vi "Untitled 1 (SubVI).vi"(7 "Comm":enum16{"Init", "Clear", "Update Data"}(ring), 8 "error in (no error)":errorcluster, 10 "Channels info":string[](array[string])=["燃烧室压力1\n[MPa]", "燃烧室压力1\n[MPa]"], 11 "ML Ref":refnum<vi>) -> (0 "error out":errorcluster)   [LabVIEW 2016]
uses:
  <vilib>/Utility/miscctls.llb/LVRowAndColumnTypeDef.ctl
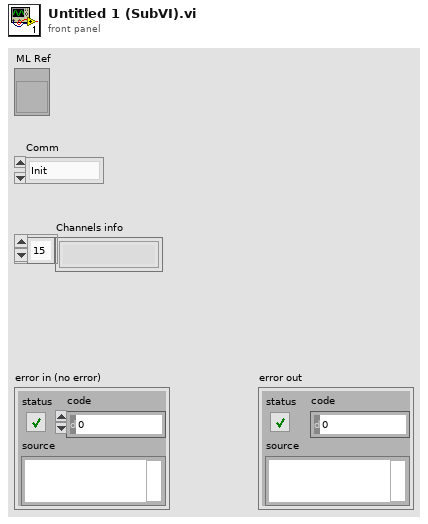
[diagram p1: front panel]
types:
  T1 = cluster{"Font Name":string, "Size":u16, "Bold":bool, "Italic":bool, "Underline":bool, "Strikeout":bool, u32}
  T2 = typedef "LVRowAndColumnTypeDef.ctl" = cluster{"Row":i32, "Column":i32}
  T3 = typedef "LVBoundsTypeDef.ctl" = cluster{"Width":u32, "Height":u32}
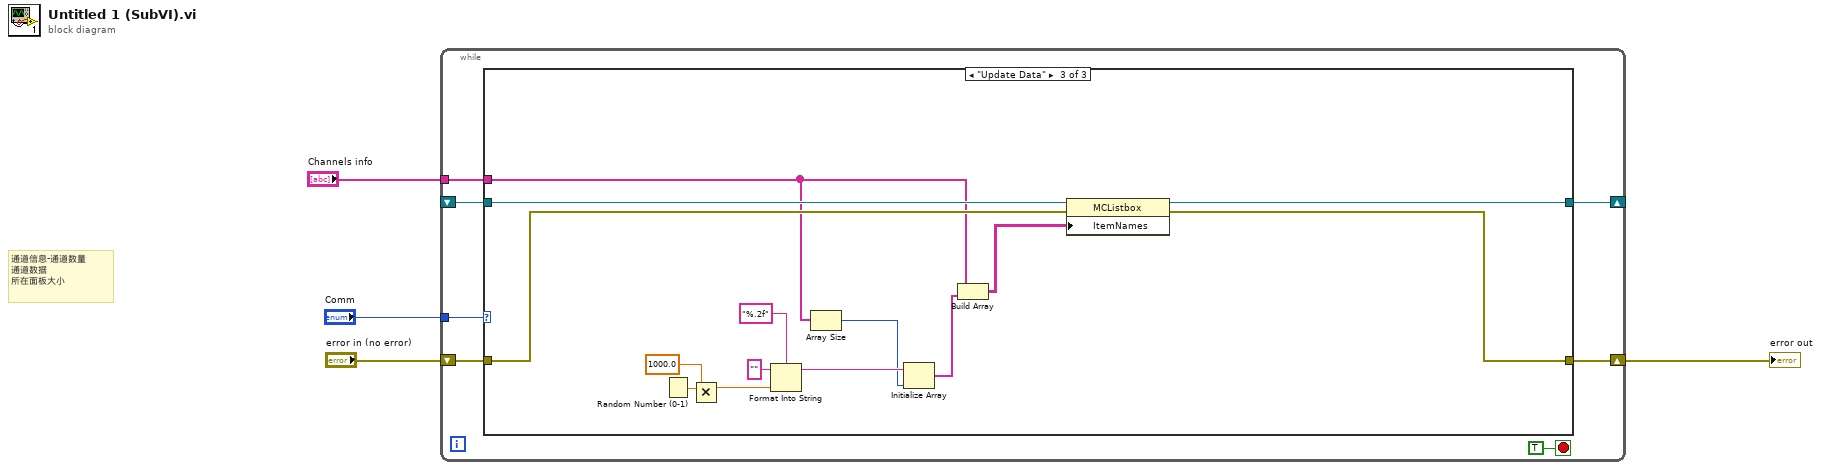
[diagram p0: block diagram]
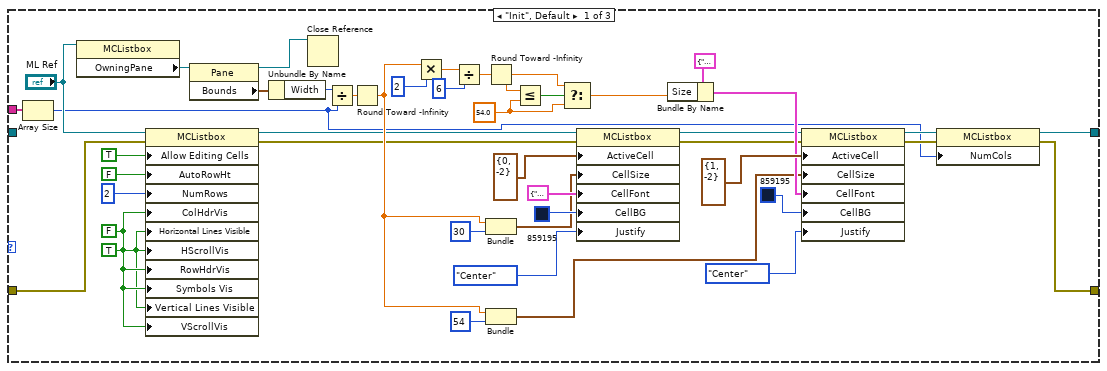
[diagram p2: hidden frame]
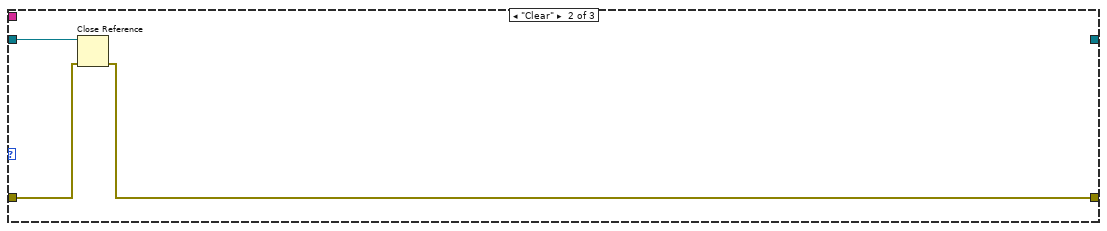
[diagram p3: hidden frame]
diagram:
  # "通道信息-通道数量\n通道数据\n所在面板大小"
  n1 = while {
    tunnel: "Comm" -> [w10]
    shift-right: [w7] -> _
    shift-left: _ -> [w6]
    shift-right: [w8] -> w2
    shift-left: "error in (no error)" -> [w9]
    tunnel: "Channels info" -> [w5]
    stop <- TRUE stop-if-true
    n2 = case shown="\"Update Data\"" w10 {
      tunnel: w9 -> [w50 w58 w72]
      tunnel: [w13 w57 w69] -> w8
      tunnel: [w15 _ w70] -> w7
      tunnel: w6 -> [_ w56 w71]
      tunnel: w5 -> [w41 _ w63]
      frame "Init", Default {
        w32 = 54.0 ("y")
        w51 = TRUE ("Visible Items:Column Headers Visible")
        w52 = FALSE ("Visible Items:Column Headers Visible")
        n3 = Array Size(array=w41) -> (size(s)=w12:i32)
        n4 = property class="MCListbox"(reference="ML Ref") -> ("OwningPane"=w39:refnum<vi>)  [unwired: 1 in, 2 out]
        n5 = property class="MCListbox"(reference="ML Ref", error in=w50, "Allow Editing Cells"=TRUE, "AutoRowHt"=FALSE ("Autosizing Row Height"), "NumRows"=u32 2 ("Number of Rows"), "ColHdrVis"=w52, "Horizontal Lines Visible"=w51, "HScrollVis"=w52, "RowHdrVis"=w52, "Symbols Vis"=w52, "Vertical Lines Visible"=w51, "VScrollVis"=w52) -> (reference out=w19:refnum<vi>, error out=w18:errorcluster)
        n6 = property class="Pane"(reference=w39) -> (reference out=w28:refnum<vi>, "Bounds"=w30:T3)  [unwired: 1 in, 1 out]
        n7 = Unbundle By Name(w30) -> ("Width"=w29:u32)
        n8 = Close Reference(reference=w28) -> ()  [unwired: 1 in, 1 out]
        n9 = Divide(x=w29, y=w12) -> (x/y=w38:dbl)
        n10 = Round Toward -Infinity(1:w38) -> (0:w21:dbl)
        n11 = Multiply(x=w21, y=u32 2) -> (x*y=w36:dbl)
        n12 = Divide(x=w36, y=u32 6) -> (x/y=w33:dbl)
        n13 = Round Toward -Infinity(1:w33) -> (0:w31:dbl)
        n14 = Bundle(w21, "Height"=u32 30) -> (w26:cluster{dbl, "Height":u32})  [unwired: 1 in]
        n15 = Bundle(w21, "Height"=u32 54) -> (w20:cluster{dbl, "Height":u32})  [unwired: 1 in]
        n16 = Less Or Equal?(x=w31, y=w32) -> (x <= y?=w34:bool)
        n17 = Select(t=w31, s=w34, f=w32) -> (s? t:f=w23:dbl)
        n18 = property class="MCListbox"(reference=w19, error in=w18, "ActiveCell"=T2 {"Row"=0, "Column"=-2} ("Active Cell:Active Cell"), "CellSize"=w26, "CellFont"=T1 {"Font Name"="Tahoma", "Size"=14, "Bold"=TRUE, "Italic"=FALSE, "Underline"=FALSE, "Strikeout"=FALSE, 16448250}, "CellBG"=u32 859195, "Justify"=enum16{"Left", "Center", "Right"}."Center" ("Active Cell:Cell Justification")) -> (reference out=w17:refnum<vi>, error out=w16:errorcluster)
        n19 = Bundle By Name(cluster=T1 {"Font Name"="Tahoma", "Size"=54, "Bold"=TRUE, "Italic"=FALSE, "Underline"=FALSE, "Strikeout"=FALSE, 7459327}, "Size"=w23) -> (w24:T1)
        n20 = property class="MCListbox"(reference=w17, error in=w16, "ActiveCell"=T2 {"Row"=1, "Column"=-2} ("Active Cell:Active Cell"), "CellSize"=w20, "CellFont"=w24, "CellBG"=u32 859195, "Justify"=enum16{"Left", "Center", "Right"}."Center" ("Active Cell:Cell Justification")) -> (reference out=w42:refnum<vi>, error out=w14:errorcluster)
        n21 = property class="MCListbox"(reference=w42, error in=w14, "NumCols"=w12) -> (reference out=w15:refnum<vi>, error out=w13:errorcluster)
      }
      frame "Clear" {
        n22 = Close Reference(reference=w56, error in (no error)=w58) -> (error out=w57:errorcluster)
      }
      frame "Update Data" {
        n23 = Random Number (0-1)() -> (number: 0 to 1=w64:dbl)
        n24 = Multiply(x=w64, y=1000.0) -> (x*y=w67:dbl)
        n25 = Format Into String(format string="%.2f", initial string="", w67) -> (resulting string=w62:string)  [unwired: 1 in, 1 out]
        n26 = Array Size(array=w63) -> (size(s)=w61:i32)
        n27 = Initialize Array(w62, w61) -> (w60:string[])
        n28 = Build Array(w63, w60) -> (w59:string[][])
        n29 = property class="MCListbox"(reference=w71, error in=w72, "ItemNames"=w59) -> (reference out=w70:refnum<vi>, error out=w69:errorcluster)
      }
    }
  }
  "error out" <- w2
